vi "setupUserEvents.vi"(8 "error in (no error)":errorcluster, 9 "UserEvents in":refnum<class "UserEvents.lvclass">, 10 "Model in":refnum<class "Model.lvclass">, 11 "Bootloader in":refnum<class "Bootloader.lvclass">) -> (0 "error out":errorcluster, 1 "UserEvents out":refnum<class "UserEvents.lvclass">, 2 "Model out":refnum<class "Model.lvclass">, 3 "Bootloader out":refnum<class "Bootloader.lvclass">)   [LabVIEW 2015, in "Bootloader.lvclass"]
uses:
  Bootloader.lvclass
  Model/Model.lvclass
  UserEvents/UserEvents.lvclass
  Model/Model.lvclass/Model.ctl
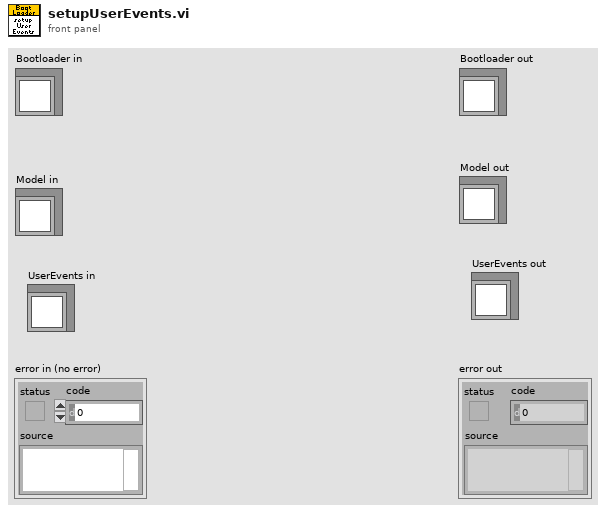
[diagram p1: front panel]
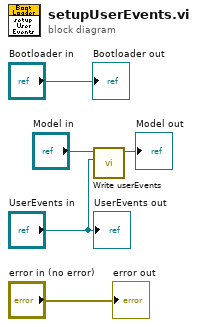
[diagram p0: block diagram]
diagram:
  n1 = call "Write userEvents.vi"("userEvents"="UserEvents in", "Model in"="Model in") -> ("Model out"=→"Model out":refnum<class "Model.lvclass">)  [unwired: 9 in]
  "error out" <- "error in (no error)"
  "Bootloader out" <- "Bootloader in"
  "UserEvents out" <- "UserEvents in"
